vi "heartbeat.vi"(8 "error in (no error)":errorcluster, 11 "tcpDevice in":refnum<class "tcpDevice.lvclass">) -> (0 "error out":errorcluster, 1 "newValue":bool, 2 "status":T1, 3 "tcpDevice out":refnum<class "tcpDevice.lvclass">, 5 "timeout?":bool)   [LabVIEW 2016, in "tcpDevice.lvclass"]
uses:
  tcpDevice.lvclass
  typedefs/deviceStatus.ctl
  typedefs/statusEnum.ctl
  tcpDevice.lvclass/tcpDevice.ctl
  deviceHeartbeat/deviceHeartbeat.lvclass
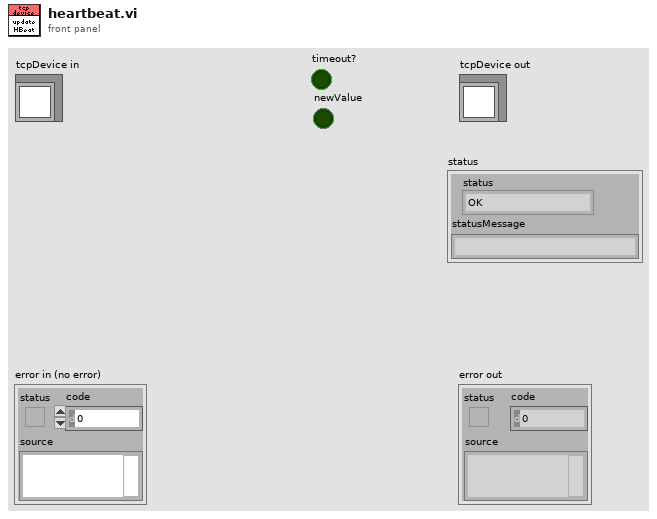
[diagram p1: front panel]
types:
  T1 = typedef "deviceStatus.ctl" = cluster{"status":T2, "statusMessage":string}
  T2 = typedef "statusEnum.ctl" = enum16{"OK", "TIMEOUT", "MSGERROR"}
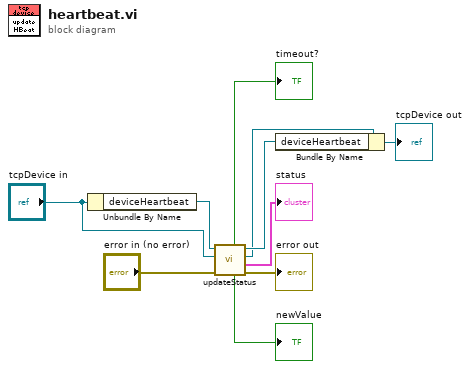
[diagram p0: block diagram]
diagram:
  n1 = Unbundle By Name("tcpDevice in") -> ("deviceHeartbeat"=w9:refnum<class "deviceHeartbeat.lvclass">)
  n2 = call "updateStatus.vi"("error in (no error)"="error in (no error)", "tcpDevice"="tcpDevice in", "deviceHeartbeat in"=w9) -> ("error out"=→"error out":errorcluster, "status"=→"status":T1, "tcpDevice out"=w6:refnum<class "tcpDevice.lvclass">, "deviceHeartbeat out"=w8:refnum<class "deviceHeartbeat.lvclass">, "newValue"=→"newValue":bool, "timeout?"=→"timeout?":bool)  [unwired: 3 in]
  n3 = Bundle By Name(cluster=w6, "deviceHeartbeat"=w8) -> (→"tcpDevice out":refnum<class "tcpDevice.lvclass">)
